vi "LJUD_GetDriverVersion.vi"() -> (3 "Driver Version":dbl format="%.2f")   [LabVIEW 2021]
doc: "Returns the version number of this Windows LabJack driver.\n\nDocumented in Section 4.2 of the device's datasheet."
uses:
  labjackud.dll
panel:
  # "Returns the version number of this Windows LabJack driver.\n\nDocumented in Section 4.2 of the device's datasheet."
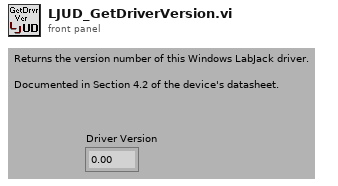
[diagram p1: front panel]
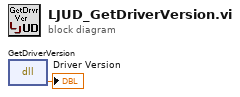
[diagram p0: block diagram]
diagram:
  n1 = dll-call lib="labjackud.dll" fn="GetDriverVersion"() -> (→"Driver Version":dbl)  [unwired: 3 in, 2 out]
